vi "cDAQ Weight Measure.vi"(5 "Offset":dbl, 7 "Truncation":i32=600, 11 "Error In":errorcluster) -> (10 "Ave in Median Range":dbl=110.07240142199429, 14 "Weight":dbl=110.06775386263871, 15 "Error Out":errorcluster)   [LabVIEW 2014]
uses:
  <vilib>/DAQmx/read.llb/DAQmx Read (Analog Wfm 1Chan NSamp).vi
  <vilib>/Analysis/NI_AALBase.lvlib
panel:
  in  "Weight Task":refnum<k21>="Weight"
  out "Unfiltered Weight":waveform(dbl)(graph)={"t0"=timestamp(0 s since 1904-01-01), "dt"=1.0, "Y"=array[3000 elements]}
  in  "Chop Width":i32=600
  in  "MA Filter Order":i32=5
  out "size(s)":i32=1800
  in  "stop":bool
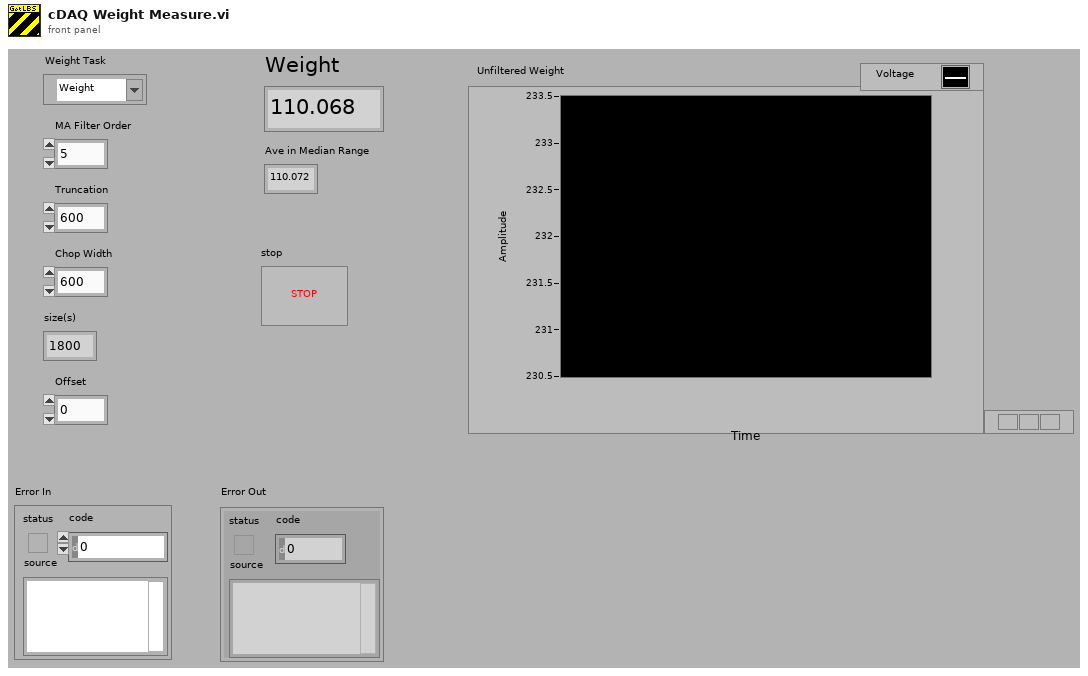
[diagram p1: front panel]
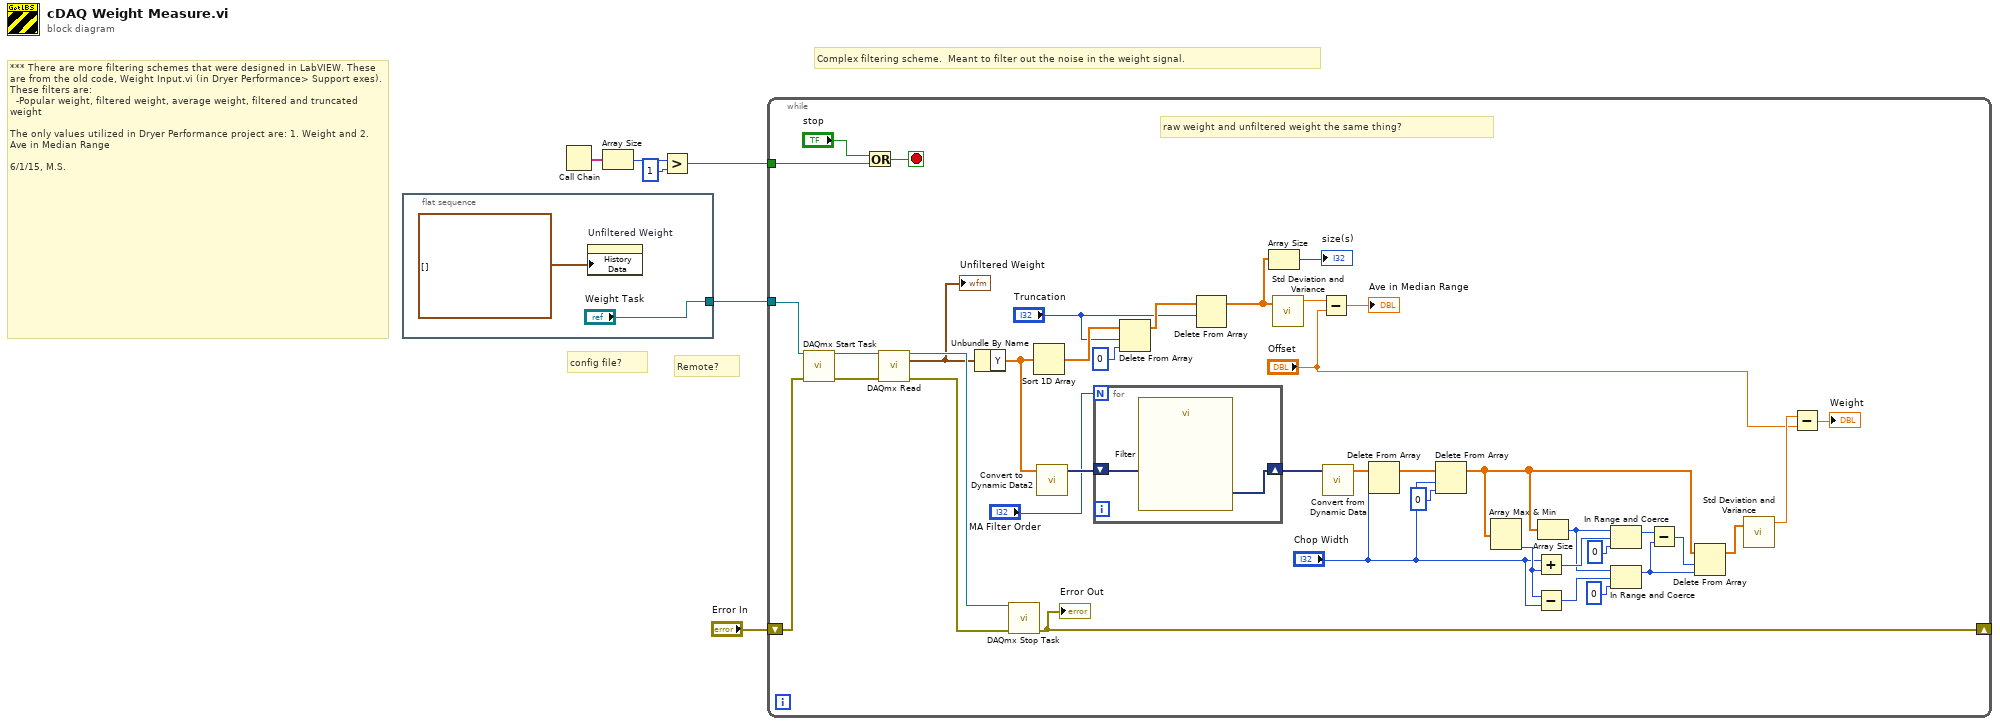
[diagram p0: block diagram]
diagram:
  # "*** There are more filtering schemes that were designed in LabVIEW. These are from the old code, Weight Input.vi (in Dryer Performance> Support exes).\nThese filters are:\n  -Popular weight, filtered weight, average weight, filtered and truncated weight\n\nThe only values utilized in Dryer Performance project are: 1. Weight and 2. Ave in Median Range\n\n6/1/15, M.S."
  # "config file?"
  # "Complex filtering scheme.  Meant to filter out the noise in the weight signal."
  # "Remote?"
  n1 = flat-sequence {
    tunnel: ["Weight Task"] -> w6
    frame #0 {
      n2 = property on="Unfiltered Weight" class="WFChart (strict)"("History Data"=waveform(dbl)[] []) -> ()  [unwired: 2 in, 2 out]
    }
  }
  n3 = Call Chain() -> (call chain=w4:string[])
  n4 = Array Size(array=w4) -> (size(s)=w3:i32)
  n5 = Greater?(x=w3, y=1) -> (0:w1:bool)
  n6 = while {
    tunnel: w6 -> [w48]
    shift-right: [w43] -> _
    shift-left: "Error In" -> [w46]
    tunnel: w1 -> [w40]
    stop <- w41 stop-if-true
    # "raw weight and unfiltered weight the same thing?"
    n7 = call <vilib>:"DAQmx Start Task.vi"("task/channels in"=w48, "error in"=w46) -> ("task out"=w47:refnum<k21>, "error out"=w45:errorcluster)  [unwired: 12 in]
    n8 = Or(x="stop", y=w40) -> (x .or. y?=w41:bool)
    n9 = call-poly <vilib>:"DAQmx Read.vi"("task/channels in"=w47, "error in"=w45) -> ("task out"=w42:refnum<k21>, "data"=w9:waveform(dbl), "error out"=w44:errorcluster)  [unwired: 11 in]
    "Unfiltered Weight" <- w9
    n10 = Unbundle By Name(w9) -> ("Y"=w19:dbl[])
    n11 = call <vilib>:"DAQmx Stop Task.vi"("task/channels in"=w42, "error in"=w44) -> ("error out"=w43:errorcluster)  [unwired: 12 in, 1 out]
    "Error Out" <- w43
    n12 = Sort 1D Array(array=w19) -> (sorted array=w39:dbl[])
    n13 = call "Convert to Dynamic Data2"("Array"=w19) -> ("Dynamic Data Type"=w31:dynamicdata)  [unwired: 3 in]
    n14 = for {
      N: "MA Filter Order" -> [_]
      shift-right: [w51] -> w29
      shift-left: w31 -> [w50]
      n15 = call "Filter"("Signal"=w50) -> ("Filtered Signal"=w51:dynamicdata)  [unwired: 9 in, 1 out]
    }
    n16 = Delete From Array(array=w39, length="Truncation", index=0) -> (array with subset deleted=w37:dbl[])  [unwired: 1 out]
    n17 = Delete From Array(array=w37, length="Truncation") -> (array with subset deleted=w35:dbl[])  [unwired: 1 in, 1 out]
    n18 = Array Size(array=w35) -> (size(s)=→"size(s)":i32)
    n19 = call <vilib>:"Std Deviation and Variance.vi"("X"=w35) -> ("mean"=w33:dbl)  [unwired: 1 in, 2 out]
    n20 = Subtract(x=w33, y="Offset") -> (x-y=→"Ave in Median Range":dbl)
    n21 = call "Convert from Dynamic Data"("Dynamic Data Type"=w29) -> ("Array"=w18:dbl[])  [unwired: 3 in]
    n22 = Delete From Array(array=w18, length="Chop Width") -> (array with subset deleted=w17:dbl[])  [unwired: 1 in, 1 out]
    n23 = Delete From Array(array=w17, length="Chop Width", index=0) -> (array with subset deleted=w14:dbl[])  [unwired: 1 out]
    n24 = Array Max & Min(array=w14) -> (min index (indices)=w28:i32)  [unwired: 3 out]
    n25 = Add(x="Chop Width", y=w28) -> (x+y=w27:i32)
    n26 = Subtract(x=w28, y="Chop Width") -> (x-y=w24:i32)
    n27 = Array Size(array=w14) -> (size(s)=w23:i32)
    n28 = In Range and Coerce(upper limit=w23, x=w27, lower limit=0) -> (coerced(x)=w22:i32)  [unwired: 1 out]
    n29 = In Range and Coerce(upper limit=w23, x=w24, lower limit=0) -> (coerced(x)=w21:i32)  [unwired: 1 out]
    n30 = Subtract(x=w22, y=w21) -> (x-y=w20:i32)
    n31 = Delete From Array(array=w14, length=w20, index=w21) -> (array with subset deleted=w13:dbl[])  [unwired: 1 out]
    n32 = call <vilib>:"Std Deviation and Variance.vi"("X"=w13) -> ("mean"=w12:dbl)  [unwired: 1 in, 2 out]
    n33 = Subtract(x=w12, y="Offset") -> (x-y=→"Weight":dbl)
  }
